vi "Test Create Channel Buffer.vi"(11 "Test Case In":refnum<class "Test BufferLossless.lvclass">) -> (0 "error out":errorcluster, 3 "Test Case Out":refnum<class "Test BufferLossless.lvclass">)   [LabVIEW 2024, in "Test BufferLossless.lvclass"]
uses:
  Test BufferLossless.lvclass
  C:/Program Files/National Instruments/LabVIEW 2024/vi.lib/Astemes/LUnit/Test Case.lvclass
  Devices/Buffers/BufferLossless/BufferLossless.lvclass
  <vilib>/Astemes/LUnit/Test Case.lvclass/Test Case.ctl
  <vilib>/Astemes/LUnit/Append Pass Result.vi
  <vilib>/Astemes/LUnit/Append Fail Result.vi
  <vilib>/Astemes/LUnit/Run In UI.vi
  <vilib>/Utility/error.llb/Clear Errors.vi
  <vilib>/Astemes/LUnit/Test Case.lvclass
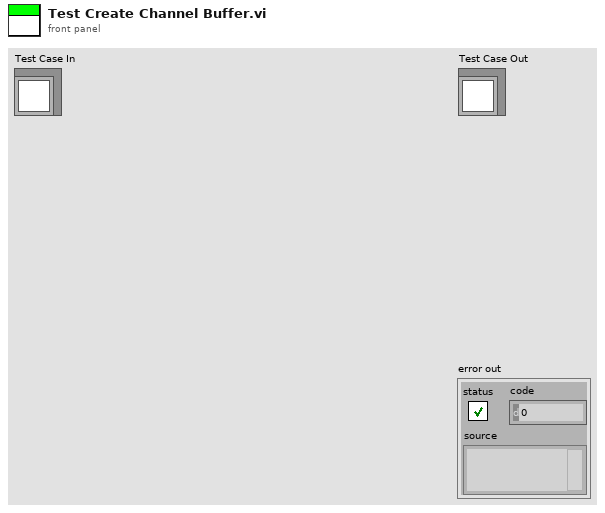
[diagram p1: front panel]
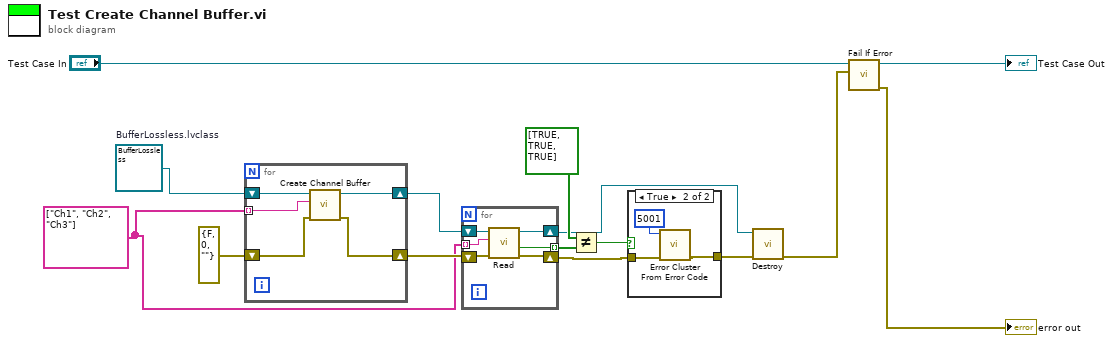
[diagram p0: block diagram]
diagram:
  w8 = string[] ["Ch1", "Ch2", "Ch3"]
  w12 = refnum<class "BufferLossless.lvclass"> refnum  # BufferLossless.lvclass
  n1 = for {
    shift-right: [w16] -> w10
    shift-left: errorcluster {"status"=FALSE, "code"=0, "source"=""} ("error in (no error)") -> [w19]
    tunnel: w8 -> [w18] mode=indexing
    shift-right: [w17] -> w9
    shift-left: w12 -> [w20]
    n2 = call "Create Channel Buffer.vi"("error in"=w19, "Channel"=w18, "BufferLossless in"=w20) -> ("error out"=w16:errorcluster, "BufferLossless out"=w17:refnum<class "BufferLossless.lvclass">)  [unwired: 7 in]
  }
  n3 = for {
    tunnel: w8 -> [w24] mode=indexing
    shift-right: [w23] -> w2
    shift-left: w9 -> [w25]
    shift-right: [w22] -> w6
    shift-left: w10 -> [w26]
    tunnel: [w21] -> w7 mode=indexing
    n4 = call "Read.vi"("error in"=w26, "Channel"=w24, "BufferLossless in"=w25) -> ("error out"=w22:errorcluster, "empty?"=w21:bool, "BufferLossless out"=w23:refnum<class "BufferLossless.lvclass">)  [unwired: 5 in, 1 out]
  }
  n5 = Not Equal?(x=bool[] [TRUE, TRUE, TRUE], y=w7) -> (x != y?=w4:bool)
  n6 = case shown="True" w4 {
    tunnel: w6 -> [w27 w30]
    tunnel: [w27 w29] -> w3
    frame False {
    }
    frame True {
      n7 = call <vilib>:"Error Cluster From Error Code.vi"("error in (no error)"=w30, "error code (0)"=5001) -> ("error out"=w29:errorcluster)  [unwired: 7 in]
    }
  }
  n8 = call "Destroy.vi"("error in"=w3, "BufferLossless in"=w2) -> ("error out"=w1:errorcluster)  [unwired: 8 in, 1 out]
  n9 = call <vilib>:"Fail If Error.vi"("Assert error"=w1, "LUnit Test Case In"="Test Case In") -> ("error out"=→"error out":errorcluster, "LUnit Test Case Out"=→"Test Case Out":refnum<class "Test BufferLossless.lvclass">)  [unwired: 8 in]
